vi "ACT_LabVIEW4_Task1A_Team072.vi"(10 "r, radius (m)":dbl, 11 "m, mass (kg)":dbl) -> (3 "g, acceleration due to gravity":dbl)   [LabVIEW 2016]
uses:
  <vilib>/express/express arith-compare/Formula/XNode/ExpressFormulaBlockNode.xnode
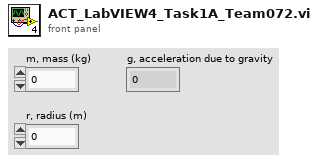
[diagram p1: front panel]
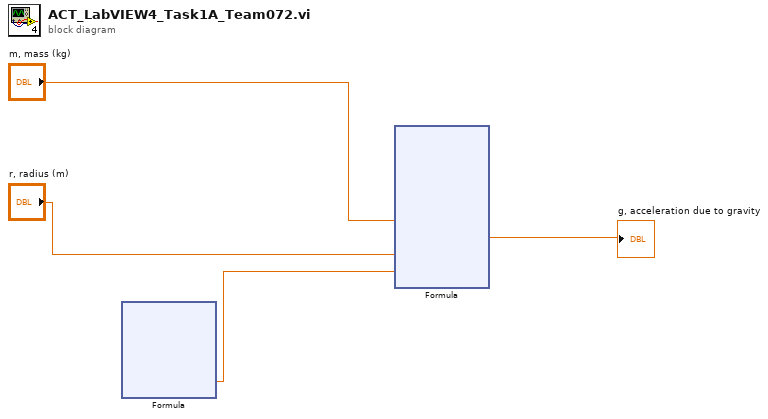
[diagram p0: block diagram]
diagram:
  n1 = xnode "Formula"() -> ("Result"=w1:dbl)  [unwired: 1 in, 1 out]
  n2 = xnode "Formula"("m"="m, mass (kg)", "r"="r, radius (m)", "G"=w1) -> ("Result"=→"g, acceleration due to gravity":dbl)  [unwired: 1 in, 1 out]
